vi "AnglePidController (SubVI).vi"(4 "Sum Error":dbl, 5 "Previous Error":dbl, 6 "Wall Tracking Boolean":bool, 7 "Robot Width (m)":dbl, 10 "Desired Speed (m|s)":dbl, 11 "PID Setpoint [Wall Distance (m) OR Heading (deg)]":dbl) -> (0 "Velocity Right (m|s)":dbl, 1 "Sum For Shift Register":dbl, 2 "Current Error":dbl, 3 "Velocity Left (m|s)":dbl)   [LabVIEW 2017]
panel:
  in  "Angle D":dbl=0.0001
  in  "Angle I":dbl
  in  "Angle_P":dbl=0.002
  out "Angle Error":dbl(graph)
  out "Plot for Kd":dbl(graph)
  in  "kD":dbl=-0.1
  in  "kI":dbl
  in  "kP":dbl=0.12
  out "PID OUTPUT":dbl(graph)
  out "Current Error":dbl(graph)
  out "Shared Variable Heading (deg)":dbl
  out "Robot Heading (deg)":dbl
  in  "Right Encoder Distance (m)":dbl
  in  "Left Encoder Distance (m)":dbl
  # "VI Name: AnglePidController (SubVI).vi\nAuthor: Steven Lee\n\nThis SubVI takes in the Encoder Count values and provide PID control for the robot's heading.\n\nInput: Theta (Desired Angle), v0 (Desired Velocity)\nOutput: v_r (right wheel velocity), v_l (left wheel velocity)"
  # "Known working parameters\nP: 0.12\nI: 0\nD: -0.1"
  # "settle with the following parameters for now:\n\nP = 0.002\nI = 0\nD = 0.0001"
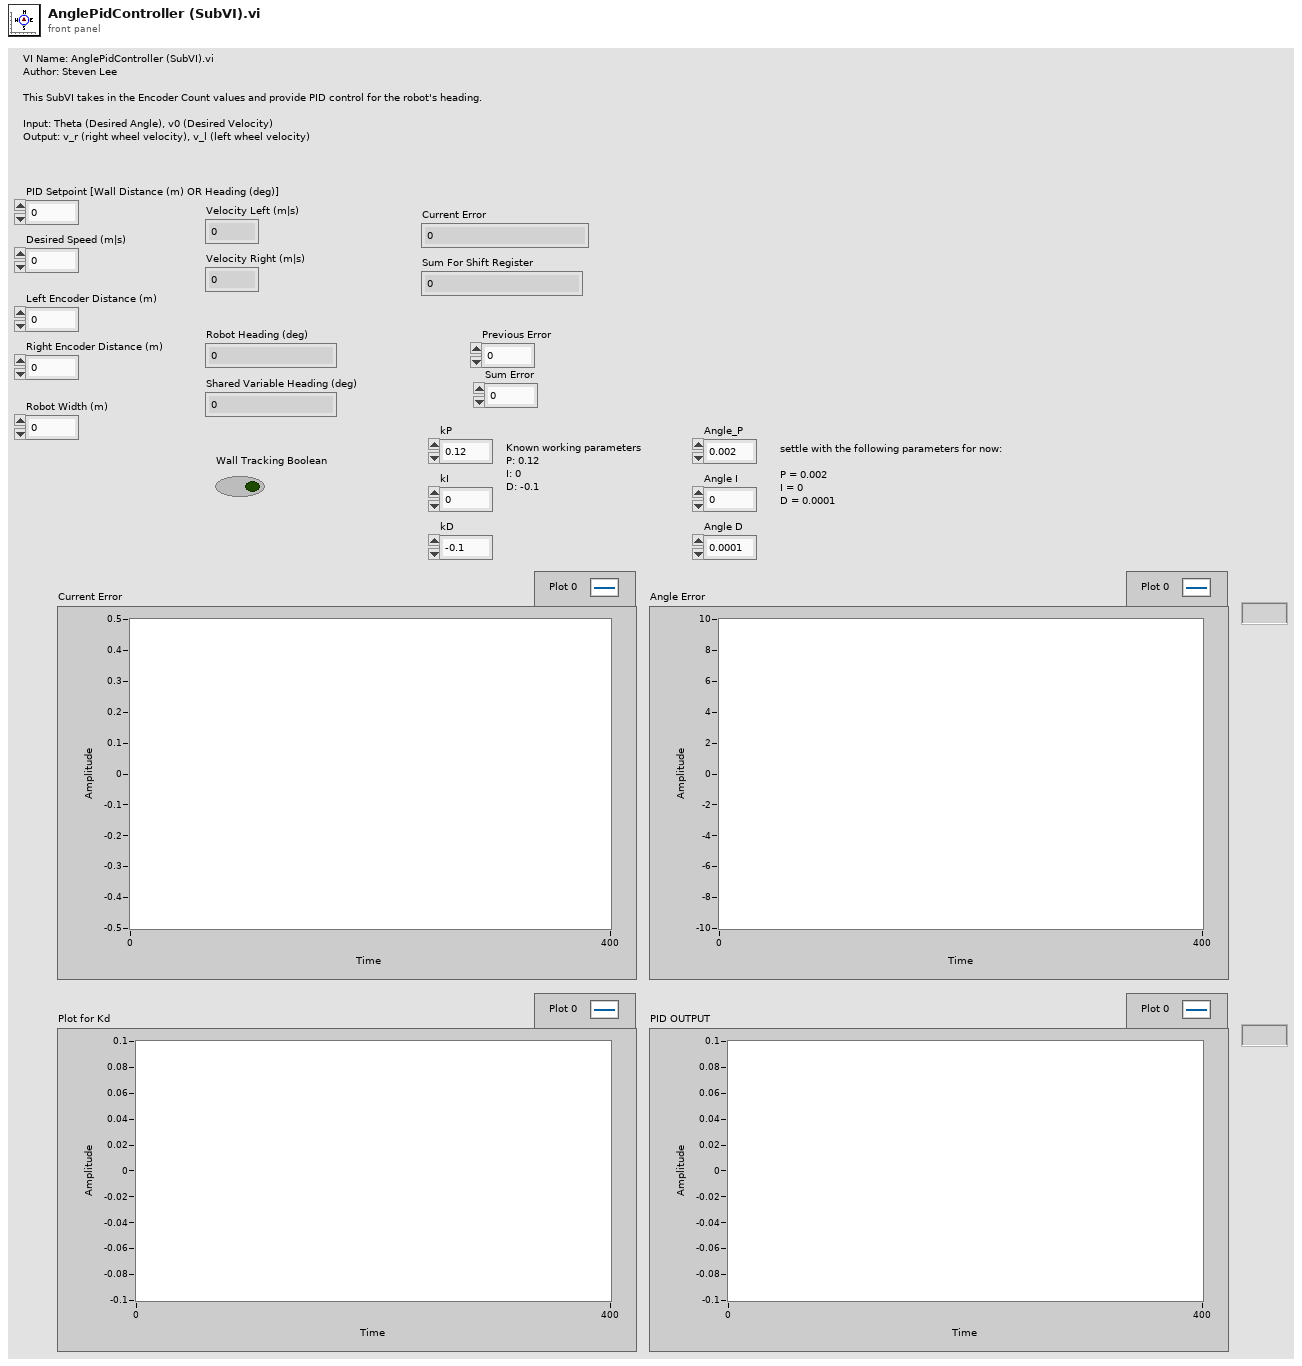
[diagram p1: front panel]
types:
  T1 = cluster{"proportional gain (Kc)":dbl, "integral time (Ti, min)":dbl, "derivative time (Td, min)":dbl}
  T2 = cluster{"Angle_P":dbl, "Angle I":dbl, "Angle D":dbl}
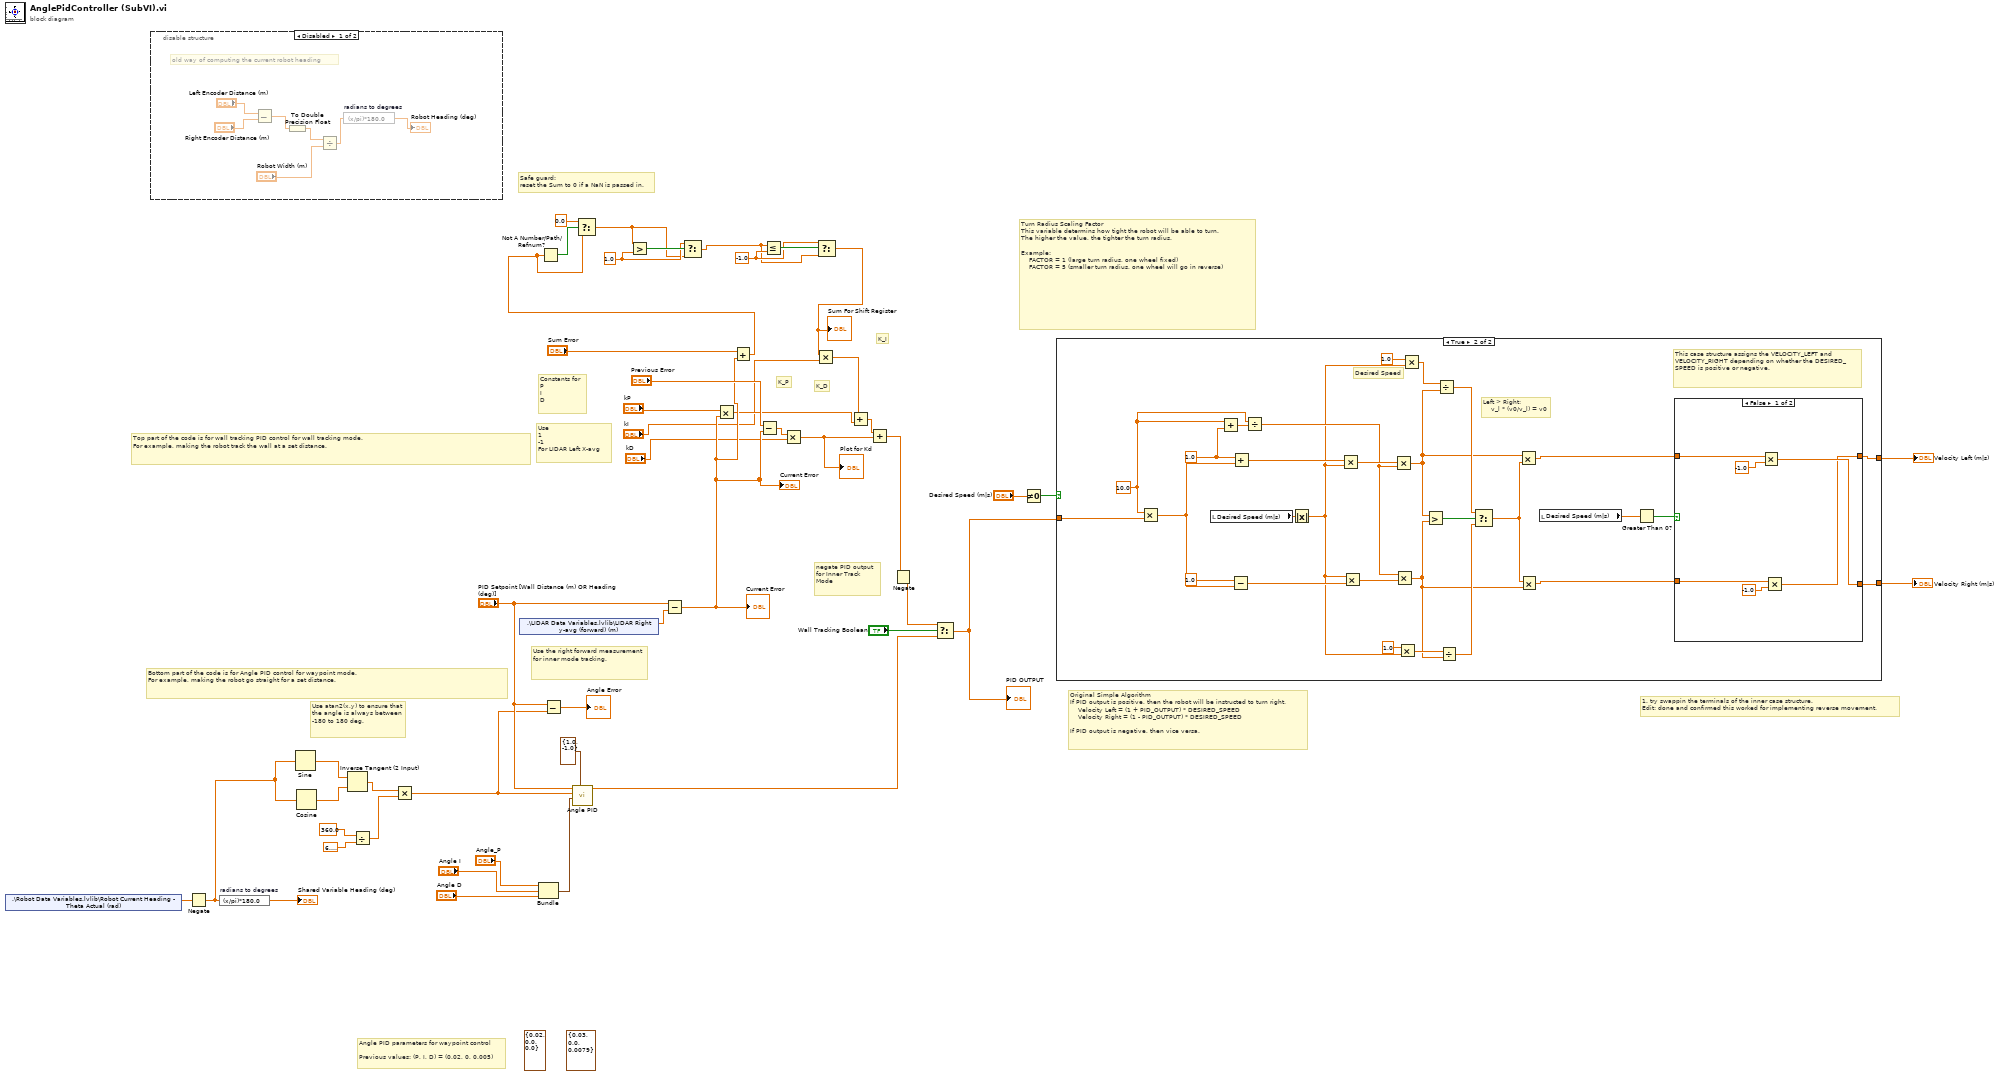
[diagram p0: block diagram]
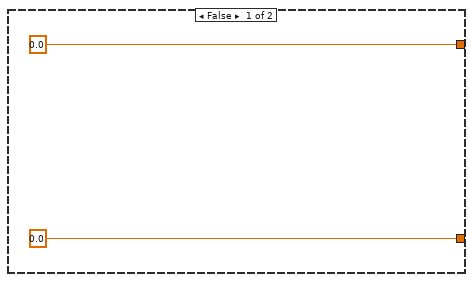
[diagram p3: hidden frame]
diagram:
  (unwired) T1 {"proportional gain (Kc)"=0.03, "integral time (Ti, min)"=0.0, "derivative time (Td, min)"=0.0079} ("PID gains")
  w29 = -1.0 ("y")
  w18 = 1.0 ("y")
  (unwired) T1 {"proportional gain (Kc)"=0.02, "integral time (Ti, min)"=0.0, "derivative time (Td, min)"=0.0} ("PID gains")
  # "Safe guard:\nreset the Sum to 0 if a NaN is passed in."
  # "Use the right forward measurement for inner mode tracking."
  # "negate PID output for Inner Track Mode"
  # "Top part of the code is for wall tracking PID control for wall tracking mode.\nFor example, making the robot track the wall at a set distance."
  # "Bottom part of the code is for Angle PID control for waypoint mode.\nFor example, making the robot go straight for a set distance."
  # "K_I"
  # "K_P"
  # "K_D"
  # "Constants for\nP\nI\nD"
  # "Angle PID parameters for waypoint control\n\nPrevious values: (P, I, D) = (0.02, 0, 0.005)"
  # "Use atan2(x,y) to ensure that the angle is always between -180 to 180 deg."
  # "Use \n1\n-1\nFor LIDAR Left X-avg"
  # "Turn Radius Scaling Factor\nThis variable determins how tight the robot will be able to turn.\nThe higher the value, the tighter the turn radius.\n\nExample:\n    FACTOR = 1 (large turn radius, one wheel fixed)\n    FACTOR = 5 (smaller turn radius, one wheel will go in reverse)"
  # "1. try swappin the terminals of the inner case structure.\nEdit: done and confirmed this worked for implementing reverse movement."
  # "Original Simple Algorithm\nIf PID output is positive, then the robot will be instructed to turn right.\n    Velocity Left = (1 + PID_OUTPUT) * DESIRED_SPEED\n    Velocity Right = (1 - PID_OUTPUT) * DESIRED_SPEED\n\nIf PID output is negative, then vice versa."
  n1 = shared-variable ".\\Robot Data Variables.lvlib\\Robot Current Heading - Theta Actual (rad)"() -> (w37:dbl)  [unwired: 1 in, 1 out]
  n2 = disable-structure shown="Disabled" {
    frame Disabled {
      # "old way of computing the current robot heading"
      n3 = Subtract(x="Left Encoder Distance (m)", y="Right Encoder Distance (m)") -> (x-y=w55:dbl)
      n4 = To Double Precision Float(number=w55) -> (double precision float=w54:dbl)
      n5 = Divide(x=w54, y="Robot Width (m)") -> (x/y=w49:dbl)
      n6 = expression code="(x/pi)*180.0" "radians to degrees"(w49) -> (→"Robot Heading (deg)":dbl)
    }
    frame Enabled {
    }
  }
  n7 = Negate(x=w37) -> (-x=w35:dbl)
  n8 = expression code="(x/pi)*180.0" "radians to degrees"(w35) -> (→"Shared Variable Heading (deg)":dbl)
  n9 = Sine(x=w35) -> (sin(x)=w43:dbl)
  n10 = Cosine(x=w35) -> (cos(x)=w42:dbl)
  n11 = Inverse Tangent (2 Input)(1:w42, 2:w43) -> (0:w40:dbl)
  n12 = Divide(x=360.0 ("y"), y=6.283185307179586) -> (x/y=w39:dbl)
  n13 = Multiply(x=w40, y=w39) -> (x*y=w11:dbl)
  n14 = shared-variable ".\\LIDAR Data Variables.lvlib\\LIDAR Right y-avg (forward) (m)"() -> (w17:dbl)  [unwired: 1 in, 1 out]
  n15 = Bundle("Angle_P"="Angle_P", "Angle I"="Angle I", "Angle D"="Angle D") -> (w6:T2)  [unwired: 1 in]
  n16 = Subtract(x="PID Setpoint [Wall Distance (m) OR Heading (deg)]", y=w11) -> (x-y=→"Angle Error":dbl)
  n17 = call "Angle PID.vi"("output range"=cluster{"output high":dbl, "output low":dbl} {"output high"=1.0, "output low"=-1.0}, "PID gains"=w6, "process variable"=w11, "setpoint"="PID Setpoint [Wall Distance (m) OR Heading (deg)]") -> ("output"=w14:dbl)  [unwired: 6 in, 1 out]
  n18 = Subtract(x="PID Setpoint [Wall Distance (m) OR Heading (deg)]", y=w17) -> (x-y=w32:dbl)
  "Current Error" <- w32
  "Current Error" <- w32
  n19 = Multiply(x="kP", y=w32) -> (x*y=w24:dbl)
  n20 = Add(x="Sum Error", y=w32) -> (x+y=w2:dbl)
  n21 = Not A Number/Path/Refnum?(number/path/refnum=w2) -> (NaN/Path/Refnum?=w4:bool)
  n22 = Select(t=0.0, s=w4, f=w2) -> (s? t:f=w1:dbl)
  n23 = Greater?(x=w1, y=w18) -> (0:w31:bool)
  n24 = Select(t=w18, s=w31, f=w1) -> (s? t:f=w28:dbl)
  n25 = Subtract(x="Previous Error", y=w32) -> (x-y=w33:dbl)
  n26 = Less Or Equal?(x=w28, y=w29) -> (x <= y?=w30:bool)
  n27 = Multiply(x=w33, y="kD") -> (x*y=w19:dbl)
  "Plot for Kd" <- w19
  n28 = Select(t=w29, s=w30, f=w28) -> (s? t:f=w26:dbl)
  "Sum For Shift Register" <- w26
  n29 = Multiply(x=w26, y="kI") -> (x*y=w23:dbl)
  n30 = Add(x=w23, y=w24) -> (x+y=w25:dbl)
  n31 = Add(x=w25, y=w19) -> (x+y=w15:dbl)
  n32 = Negate(x=w15) -> (-x=w5:dbl)
  n33 = Select(t=w5, s="Wall Tracking Boolean", f=w14) -> (s? t:f=w13:dbl)
  "PID OUTPUT" <- w13
  n34 = Not Equal To 0?(x="Desired Speed (m|s)") -> (x != 0?=w44:bool)
  n35 = case shown="True" w44 {
    tunnel: w13 -> [_ w71]
    tunnel: [0.0 w59] -> w47
    tunnel: [0.0 w58] -> w46
    frame False {
    }
    frame True {
      w67 = 10.0 ("x")
      w69 = 1.0 ("x")
      # "This case structure assigns the VELOCITY_LEFT and VELOCITY_RIGHT depending on whether the DESIRED_SPEED is positive or negative."
      # "Desired Speed"
      # "Left > Right: \n    v_l * (v0/v_l) = v0"
      n36 = Multiply(x=w67, y=w71) -> (x*y=w70:dbl)
      n37 = local read "Desired Speed (m|s)"() -> (w65:dbl)
      n38 = Add(x=w67, y=w69) -> (x+y=w68:dbl)
      n39 = Subtract(x=1.0, y=w70) -> (x-y=w84:dbl)
      n40 = Add(x=w69, y=w70) -> (x+y=w85:dbl)
      n41 = Divide(x=w67, y=w68) -> (x/y=w66:dbl)
      n42 = Absolute Value(x=w65) -> (abs(x)=w64:dbl)
      n43 = Multiply(x=w85, y=w64) -> (x*y=w83:dbl)
      n44 = Multiply(x=w64, y=w84) -> (x*y=w82:dbl)
      n45 = Multiply(x=w83, y=w66) -> (x*y=w74:dbl)
      n46 = Multiply(x=w66, y=w82) -> (x*y=w73:dbl)
      n47 = Multiply(x=1.0, y=w64) -> (x*y=w77:dbl)
      n48 = Multiply(x=1.0, y=w64) -> (x*y=w79:dbl)
      n49 = Greater?(x=w74, y=w73) -> (0:w81:bool)
      n50 = Divide(x=w79, y=w74) -> (x/y=w76:dbl)
      n51 = Divide(x=w77, y=w73) -> (x/y=w75:dbl)
      n52 = Select(t=w76, s=w81, f=w75) -> (s? t:f=w72:dbl)
      n53 = Multiply(x=w74, y=w72) -> (x*y=w61:dbl)
      n54 = Multiply(x=w72, y=w73) -> (x*y=w60:dbl)
      n55 = local read "Desired Speed (m|s)"() -> (w62:dbl)
      n56 = Greater Than 0?(x=w62) -> (x > 0?=w63:bool)
      n57 = case shown="False" w63 {
        tunnel: w61 -> [w90 w94]
        tunnel: [w87 w94] -> w59
        tunnel: w60 -> [w89 w93]
        tunnel: [w88 w93] -> w58
        frame False {
          n58 = Multiply(x=w90, y=-1.0) -> (x*y=w88:dbl)
          n59 = Multiply(x=w89, y=-1.0) -> (x*y=w87:dbl)
        }
        frame True {
        }
      }
    }
  }
  "Velocity Left (m|s)" <- w47
  "Velocity Right (m|s)" <- w46
